vi "DX3003-crc16.vi"(4 "message":string) -> (1 "CRC16":string)   [LabVIEW 2015]
doc: "This VI computes a CRC16 checksum from <B>message</B>.\nFor compatibility with the MODbus protocol the hi and low bytes of the CRC are swapped."
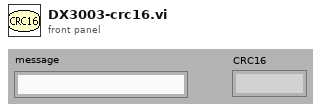
[diagram p1: front panel]
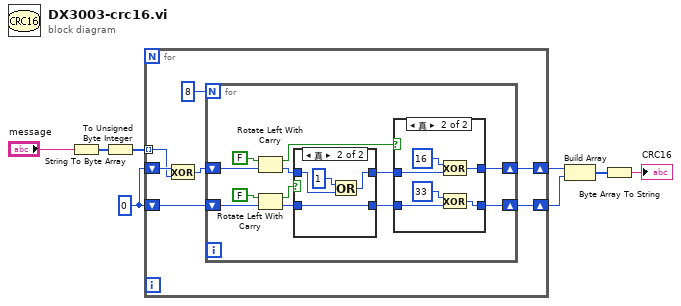
[diagram p0: block diagram]
diagram:
  w3 = u8 0
  n1 = String To Byte Array(string="message") -> (unsigned byte array=w8:u8[])
  n2 = To Unsigned Byte Integer(number=w8) -> (unsigned 8bit integer=w6:u8[])
  n3 = for {
    shift-right: [w12] -> w2
    shift-left: w3 -> [w13]
    tunnel: w6 -> [w11] mode=indexing
    shift-right: [w9] -> w1
    shift-left: w3 -> [w10]
    n4 = Exclusive Or(1:w11, 2:w13) -> (0:w14:u8)
    n5 = for {
      N: 8 -> [_]
      shift-right: [w25] -> w12
      shift-left: w14 -> [w18]
      shift-right: [w24] -> w9
      shift-left: w10 -> [w27]
      n6 = Rotate Left With Carry(2:w18, 3:FALSE ("Übertrag")) -> (0:w17:u8, 1:w20:bool)
      n7 = Rotate Left With Carry(2:w27, 3:FALSE ("Übertrag")) -> (0:w21:u8, 1:w22:bool)
      n8 = case shown="真" w22 {
        tunnel: w21 -> [w37 w38]
        tunnel: [w37 w38] -> w26
        tunnel: w17 -> [w36 w40]
        tunnel: [w36 w39] -> w16
        frame False {
        }
        frame True {
          n9 = Or(x=u8 1, y=w40) -> (x .or. y?=w39:u8)
        }
      }
      n10 = case shown="真" w20 {
        tunnel: w16 -> [w29 w34]
        tunnel: [w29 w31] -> w25
        tunnel: [w28 w30] -> w24
        tunnel: w26 -> [w28 w32]
        frame False {
        }
        frame True {
          n11 = Exclusive Or(1:w34, 2:u8 16) -> (0:w31:u8)
          n12 = Exclusive Or(1:w32, 2:u8 33) -> (0:w30:u8)
        }
      }
    }
  }
  n13 = Build Array(w2, w1) -> (w5:u8[])
  n14 = Byte Array To String(unsigned byte array=w5) -> (string=→"CRC16":string)
